vi "RandomNumber.vi"(1 "Lower Bound":dbl format="%#_13g", 3 "Upper Bound":dbl format="%#_13g") -> (0 "Value":dbl)   [LabVIEW 2014]
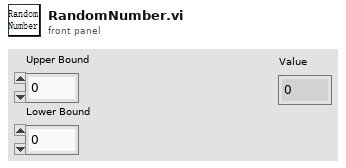
[diagram p1: front panel]
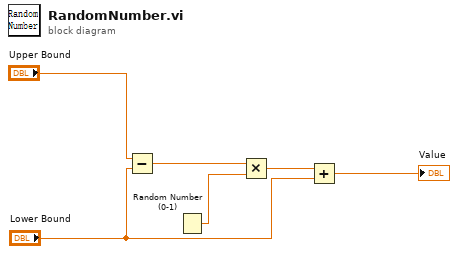
[diagram p0: block diagram]
diagram:
  n1 = Subtract(x="Upper Bound", y="Lower Bound") -> (x-y=w5:dbl)
  n2 = Random Number (0-1)() -> (number: 0 to 1=w4:dbl)
  n3 = Multiply(x=w5, y=w4) -> (x*y=w3:dbl)
  n4 = Add(x=w3, y="Lower Bound") -> (x+y=→"Value":dbl)
